vi "Scale Axis by Tick.vi"(9 "Tick Scale":dbl, 10 "Axis Focus Value":dbl, 11 "GraphScale in":refnum<vi>) -> ()   [LabVIEW 2021, in "ScrollZoomGraphChart.lvclass"]
uses:
  ScrollZoomGraphChart.lvclass
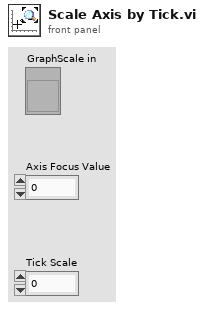
[diagram p1: front panel]
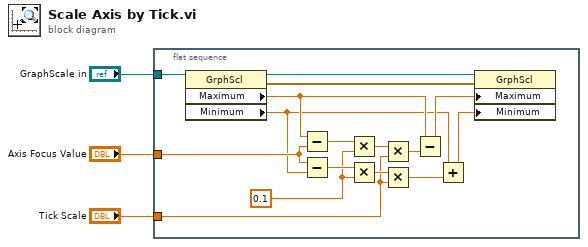
[diagram p0: block diagram]
diagram:
  n1 = flat-sequence {
    tunnel: "Axis Focus Value" -> [w19]
    tunnel: "Tick Scale" -> [w12]
    tunnel: "GraphScale in" -> [w5]
    frame #0 {
      w14 = 0.1 ("y")
      n2 = property class="GrphScl"(reference=w5) -> (reference out=w18:refnum<vi>, error out=w4:errorcluster, "Maximum"=w10:dbl, "Minimum"=w7:dbl)  [unwired: 1 in]
      n3 = Subtract(x=w10, y=w19) -> (x-y=w17:dbl)
      n4 = Subtract(x=w19, y=w7) -> (x-y=w15:dbl)
      n5 = Multiply(x=w17, y=w14) -> (x*y=w16:dbl)
      n6 = Multiply(x=w15, y=w14) -> (x*y=w13:dbl)
      n7 = Multiply(x=w16, y=w12) -> (x*y=w8:dbl)
      n8 = Multiply(x=w13, y=w12) -> (x*y=w11:dbl)
      n9 = Subtract(x=w10, y=w8) -> (x-y=w9:dbl)
      n10 = Add(x=w7, y=w11) -> (x+y=w6:dbl)
      n11 = property class="GrphScl"(reference=w18, error in=w4, "Maximum"=w9, "Minimum"=w6) -> ()  [unwired: 2 out]
    }
  }
